vi "SwissSPAD Live_Get First Event.vi"(5 "SS2 Q Element":T2[](array[typedef])) -> (0 "Data":variant, 1 "SS2 Q Event":T1=enum."Idle", 2 "SS2 Q Elements":T2[](array[typedef]))   [LabVIEW 2021]
uses:
  SwissSPAD Live_Q [Element].ctl
  SwissSPAD Live_Q Event List.ctl
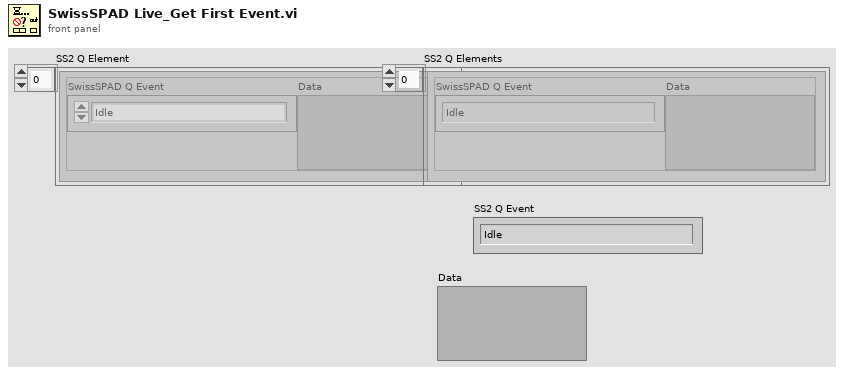
[diagram p1: front panel]
types:
  T1 = typedef "SwissSPAD Live_Q Event List.ctl" = enum16{"---- UI ----", "Idle", "Initialization", "Init FPGA(s)", "Init Top FPGA (deprecated)", "FPGA(s) Status", "Top FPGA Status (deprecated)", "Reset FPGA(s)", "Reset Top FPGA (deprecated)", "Refresh Display Image", "Quit", "---- DAQ ----", "Start Recording", "Start Live Acquisition", "Initialize Recording Mode", "Initialize FPGA (Live Mode)", "Get Image Set", "Get Single Image", "Update Image Display", "Stop Live Acquisition", "Stop Data Recording", "Stop Data Saving", "---- Image ----", "Copy Data to Clipboard", "Set Image Palette", "Save Displayed Image with Overlay", "Save Image Data as TIFF"}
  T2 = typedef "SwissSPAD Live_Q [Element].ctl" = cluster{"SwissSPAD Q Event":T1, "Data":variant}
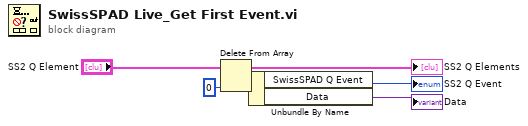
[diagram p0: block diagram]
diagram:
  n1 = Delete From Array(array="SS2 Q Element", index=0) -> (deleted portion=w6:T2, array with subset deleted=→"SS2 Q Elements":T2[])  [unwired: 1 in]
  n2 = Unbundle By Name(w6) -> ("SwissSPAD Q Event"=→"SS2 Q Event":T1, "Data"=→"Data":variant)
